vi "Test Spectrometer.vi"() -> ()   [LabVIEW 2014]
uses:
  Spectrometer Function.ctl
  Laser Settings.ctl
  Laser.ctl
  Filter.ctl
  Grating Detector Settings.ctl
  Grating.ctl
  Detector.ctl
  Acquisition Settings.ctl
  support/Instrument Status.ctl
  Spectrometer Refnum.ctl
  Measurements/Plot Data/Optical Spectrum Plot Refnum.ctl
panel:
  in  "Instrument Status":T1=TRUE
  in  "Optical Spectrum":enum32{"Energy", "Wavelength", "Raman Shift"}(tab)
  out "Optical Spectrum vs Energy":cluster{"data":dbl[], "data":dbl[]}(graph)
  out "Optical Spectrum vs Wavelength":cluster{"data":dbl[], "data":dbl[]}(graph)
  out "Optical Spectrum vs Raman Shift":cluster{"data":dbl[], "data":dbl[]}(graph)
  in  "Path":path
  in  "Acquisition Settings":T2={"Acquisition Mode"=enum."Single Window", "Spectal Position (nm)"=480.0, "From (nm)"=632.0, "To (nm)"=1000.0, "Integration Time (s)"=3.0, "Number of Accumulations"=3, "AutoScanning"=FALSE, "Spike Removal"=FALSE}
  in  "Spectrometer Settings":T3={"Confocal Hole Size (µm)"=150.0, "Grating"=1, "Detector"=enum."InGaAs Array"} {"Grating" items=["1800 l/mm", "150 l/mm"]}
  in  "Laser Settings":T6={"Laser Wavelength"=enum."633 nm", "Neutral Density Filter"=enum."1%"}
  in  "Function":T9
  in  "stop":bool
  in  "OK Button":bool
  out "error out":errorcluster
  # "LICENSED MATERIALS – PROPERTY OF IBM\nCopyright IBM Corp. 2016,\nALL RIGHTS RESERVED"
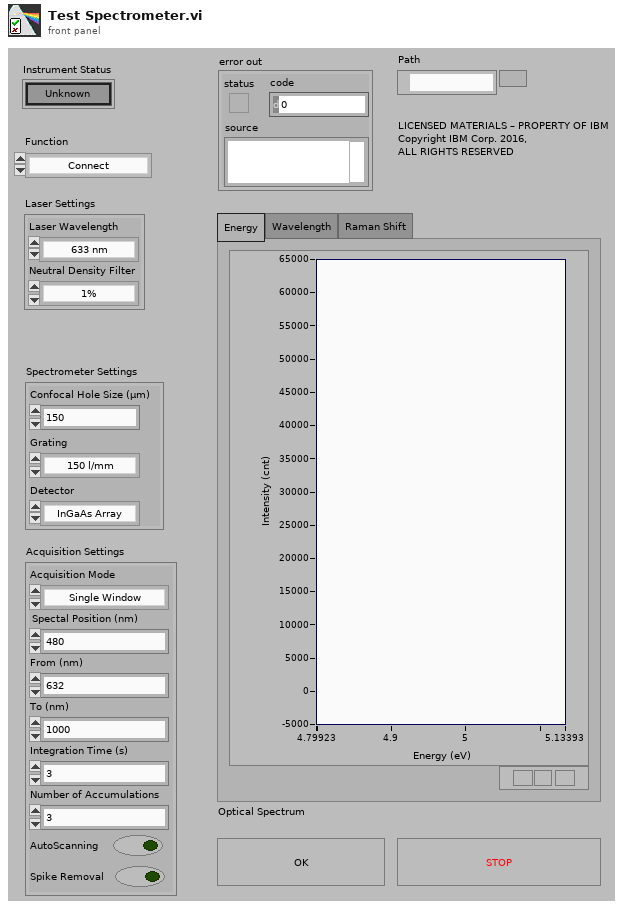
[diagram p1: front panel]
types:
  T1 = typedef "Instrument Status.ctl" = bool
  T2 = typedef "Acquisition Settings.ctl" = cluster{"Acquisition Mode":enum16{"Single Window", "Multi-Window"}, "Spectal Position (nm)":dbl, "From (nm)":dbl, "To (nm)":dbl, "Integration Time (s)":dbl, "Number of Accumulations":i32, "AutoScanning":bool, "Spike Removal":bool}
  T3 = typedef "Grating Detector Settings.ctl" = cluster{"Confocal Hole Size (µm)":dbl, "Grating":T4, "Detector":T5}
  T4 = typedef "Grating.ctl" = u16
  T5 = typedef "Detector.ctl" = enum16{"InGaAs Array", "Silicon CCD"}
  T6 = typedef "Laser Settings.ctl" = cluster{"Laser Wavelength":T7, "Neutral Density Filter":T8}
  T7 = typedef "Laser.ctl" = enum16{"633 nm", "784 nm", "532 nm", "365 nm"}
  T8 = typedef "Filter.ctl" = enum16{"100%", "50%", "25%", "10%", "1%", "0.1%", "0.01%"}
  T9 = typedef "Spectrometer Function.ctl" = enum16{"Connect", "Complete Configuration", "Get Status", "Load Configuration", "Save Configuration", "Acquire Spectrum", "Read File", "Set Laser", "Set Filter", "Set Hole", "Set Grating", "Set Grating Position", "Set Detector", "Set Acquisition Mode", "Update Refnums", "Disconnect"}
  T10 = enum8{"Enabled", "Disabled", "Disabled and Grayed Out"}
  T11 = typedef "Spectrometer Refnum.ctl" = cluster{"Instrument Status":refnum<vi>, "Optical Spectrum Plot":T12, "Laser":refnum<vi>, "Filter":refnum<vi>, "Laser ON?":refnum<vi>, "Hole":refnum<vi>, "Grating":refnum<vi>, "Detector":refnum<vi>, "Acquisition Mode":refnum<vi>, "Spectal Position":refnum<vi>, "From":refnum<vi>, "To":refnum<vi>, "Integration Time":refnum<vi>, "Accumulations":refnum<vi>, "AutoScanning":refnum<vi>, "Spike Removal":refnum<vi>, "Acquisition Mode Panel":refnum<vi>}
  T12 = typedef "Optical Spectrum Plot Refnum.ctl" = cluster{"Plot List":refnum<vi>, "Optical Spectrum vs Energy":refnum<vi>, "Optical Spectrum vs Wavelength":refnum<vi>, "Optical Spectrum vs Raman Shift":refnum<vi>, "Detector Temperature":refnum<vi>}
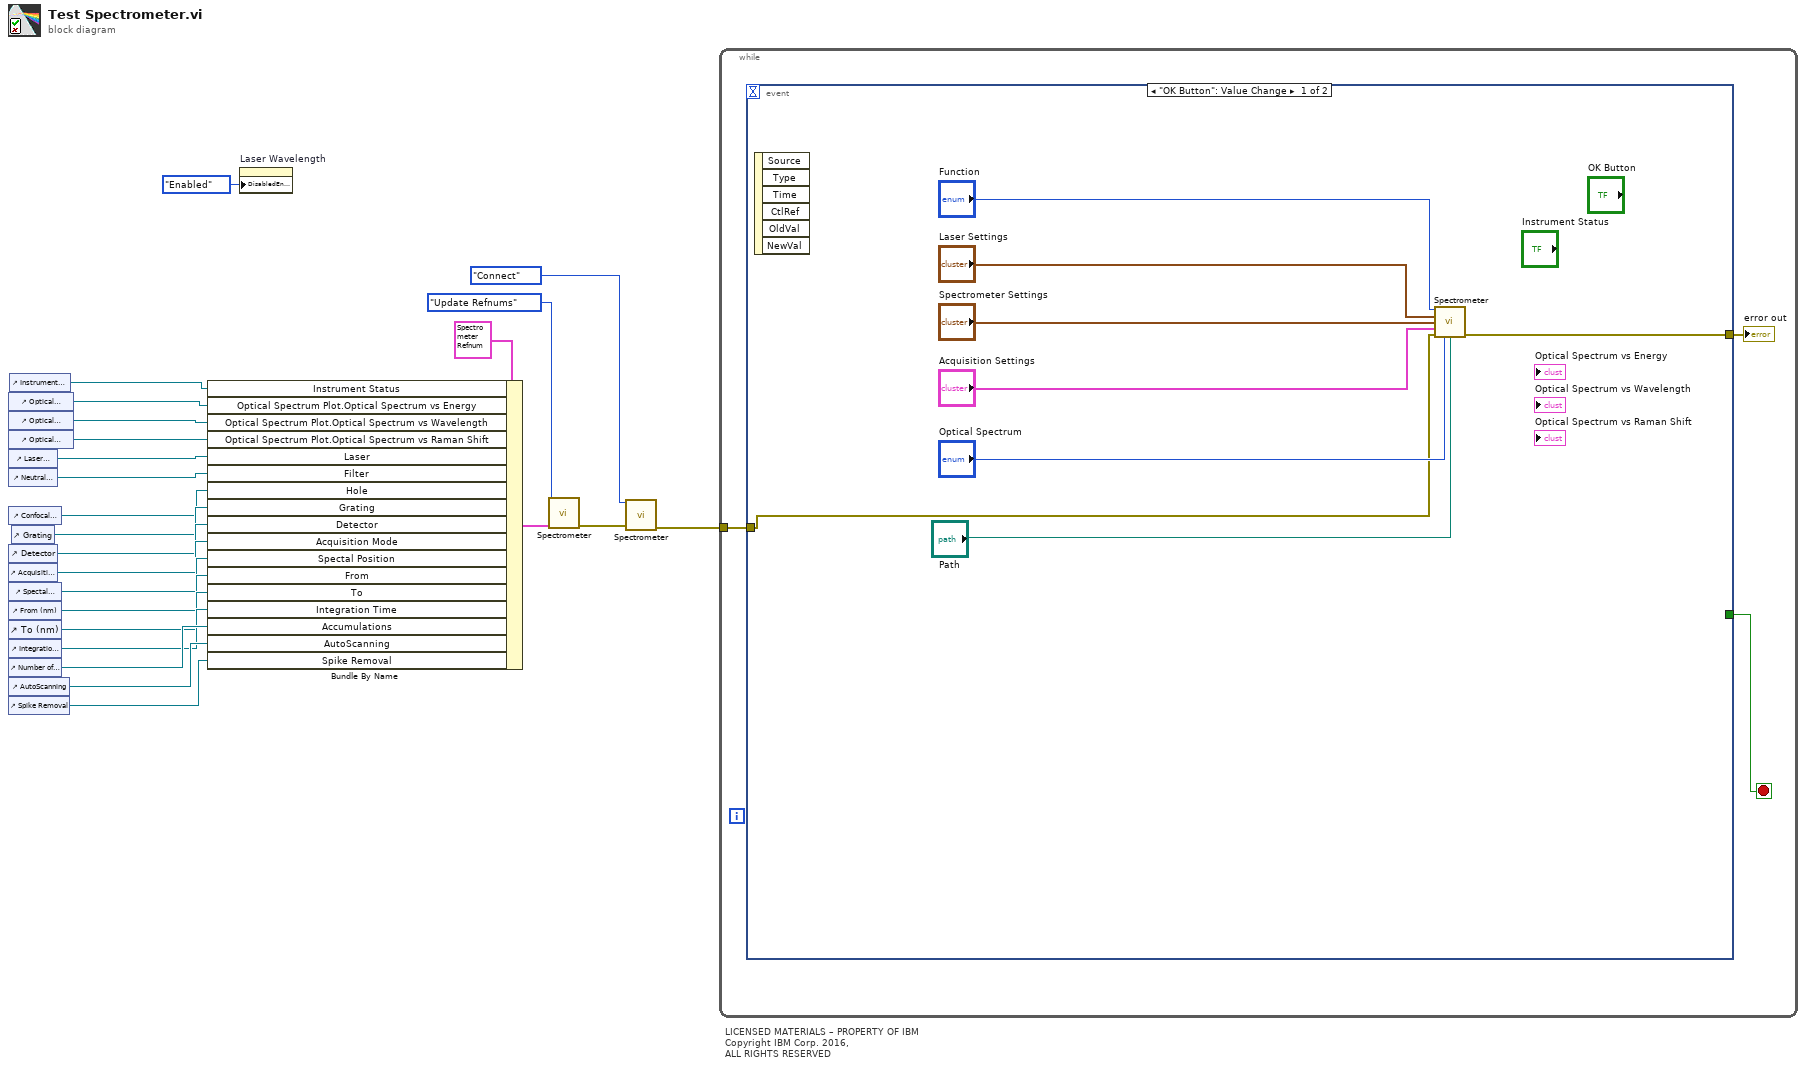
[diagram p0: block diagram]
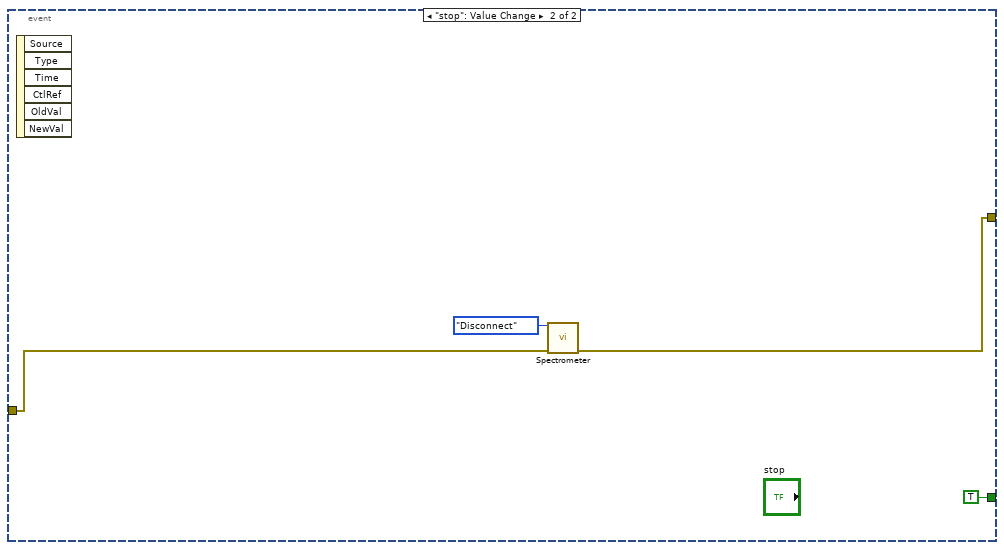
[diagram p2: hidden frame]
diagram:
  # "LICENSED MATERIALS – PROPERTY OF IBM\nCopyright IBM Corp. 2016,\nALL RIGHTS RESERVED"
  n1 = control-ref of="Optical Spectrum vs Energy"() -> (w8:refnum<vi>)
  n2 = control-ref of="Optical Spectrum vs Wavelength"() -> (w9:refnum<vi>)
  n3 = control-ref of="Optical Spectrum vs Raman Shift"() -> (w10:refnum<vi>)
  n4 = control-ref of="Laser Wavelength"() -> (w11:refnum<vi>)
  n5 = control-ref of="Neutral Density Filter"() -> (w12:refnum<vi>)
  n6 = control-ref of="Confocal Hole Size (µm)"() -> (w13:refnum<vi>)
  n7 = control-ref of="Detector"() -> (w15:refnum<vi>)
  n8 = control-ref of="Acquisition Mode"() -> (w16:refnum<vi>)
  n9 = control-ref of="Spectal Position (nm)"() -> (w17:refnum<vi>)
  n10 = control-ref of="From (nm)"() -> (w18:refnum<vi>)
  n11 = control-ref of="To (nm)"() -> (w19:refnum<vi>)
  n12 = control-ref of="Integration Time (s)"() -> (w20:refnum<vi>)
  n13 = control-ref of="Number of Accumulations"() -> (w21:refnum<vi>)
  n14 = control-ref of="AutoScanning"() -> (w22:refnum<vi>)
  n15 = control-ref of="Spike Removal"() -> (w23:refnum<vi>)
  n16 = control-ref of="Instrument Status"() -> (w24:refnum<vi>)
  n17 = control-ref of="Grating"() -> (w14:refnum<vi>)
  n18 = Bundle By Name(cluster=T11 {"Instrument Status"=refnum, "Optical Spectrum Plot"={"Plot List"=refnum, "Optical Spectrum vs Energy"=refnum, "Optical Spectrum vs Wavelength"=refnum, "Optical Spectrum vs Raman Shift"=refnum, "Detector Temperature"=refnum}, "Laser"=refnum, "Filter"=refnum, "Laser ON?"=refnum, "Hole"=refnum, "Grating"=refnum, "Detector"=refnum, "Acquisition Mode"=refnum, "Spectal Position"=refnum, "From"=refnum, "To"=refnum, "Integration Time"=refnum, "Accumulations"=refnum, "AutoScanning"=refnum, "Spike Removal"=refnum, "Acquisition Mode Panel"=refnum} ("LabramHR References"), "Instrument Status"=w24, "Optical Spectrum Plot.Optical Spectrum vs Energy"=w8, "Optical Spectrum Plot.Optical Spectrum vs Wavelength"=w9, "Optical Spectrum Plot.Optical Spectrum vs Raman Shift"=w10, "Laser"=w11, "Filter"=w12, "Hole"=w13, "Grating"=w14, "Detector"=w15, "Acquisition Mode"=w16, "Spectal Position"=w17, "From"=w18, "To"=w19, "Integration Time"=w20, "Accumulations"=w21, "AutoScanning"=w22, "Spike Removal"=w23) -> (w5:T11)
  n19 = property on="Laser Wavelength" class="Enum (strict)"("DisabledEnum"=T10."Enabled" ("Disabled")) -> ()  [unwired: 2 in, 2 out]
  n20 = call "Spectrometer.vi"("Function"=Spectrometer_Function."Update Refnums", "LabramHR References"=w5) -> ("error out"=w3:errorcluster)  [unwired: 9 in, 4 out]
  n21 = call "Spectrometer.vi"("Function"=Spectrometer_Function."Connect", "error in"=w3) -> ("error out"=w2:errorcluster)  [unwired: 9 in, 4 out]
  n22 = while {
    tunnel: w2 -> [w26]
    stop <- w27 stop-if-true
    n23 = event shown="[0] \"OK Button\": Value Change" {
      selector: _ -> [_ _]
      dyn-events: _ -> [_ _]
      timeout: _ -> [_ _]
      tunnel: [_ TRUE ("stop")] -> w27
      tunnel: w26 -> [w29 w37]
      tunnel: [w28 w36] -> w25
      event "OK Button": Value Change {
        n24 = event-data() -> ()  [unwired: 1 in, 6 out]
        n25 = call "Spectrometer.vi"("Function"="Function", "Laser Settings"="Laser Settings", "Spectrometer Settings"="Spectrometer Settings", "Acquisition Settings"="Acquisition Settings", "error in"=w29, "Optical Spectrum"="Optical Spectrum", "Path"="Path") -> ("error out"=w28:errorcluster)  [unwired: 4 in, 4 out]
      }
      event "stop": Value Change {
        n26 = event-data() -> ()  [unwired: 1 in, 6 out]
        n27 = call "Spectrometer.vi"("Function"=Spectrometer_Function."Disconnect", "error in"=w37) -> ("error out"=w36:errorcluster)  [unwired: 9 in, 4 out]
      }
    }
    "error out" <- w25
  }
